vi "Add Header.vi"(8 "error in":errorcluster, 9 "value":string, 10 "header":string, 11 "http-client in":refnum<class "http-client.lvclass">) -> (0 "error out":errorcluster, 3 "http-client out":refnum<class "http-client.lvclass">)   [LabVIEW 2025, in "http-client.lvclass"]
uses:
  http-client.lvclass
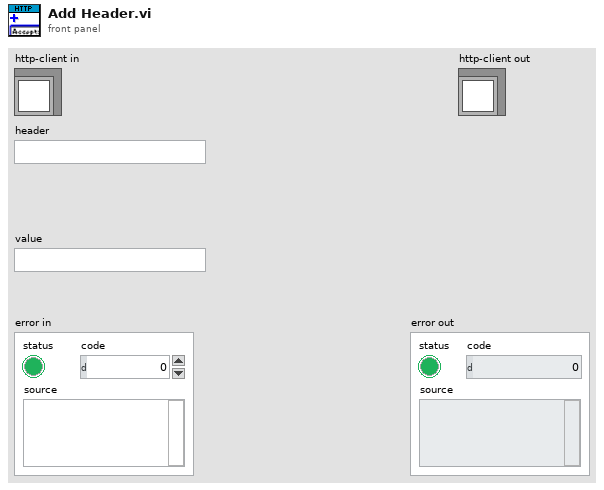
[diagram p1: front panel]
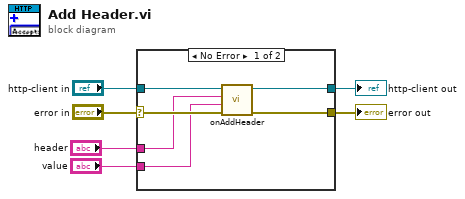
[diagram p0: block diagram]
diagram:
  n1 = case shown="No Error" "error in" {
    selector: "error in" -> [w9 w14]
    tunnel: [w10 w14] -> w5
    tunnel: [w11 w13] -> w3
    tunnel: "http-client in" -> [w12 w13]
    tunnel: "header" -> [w8 _]
    tunnel: "value" -> [w7 _]
    frame No Error {
      n2 = call-dynamic "onAddHeader.vi"("error in"=w9, "value"=w7, "header"=w8, "http-client in"=w12) -> ("error out"=w10:errorcluster, "http-client out"=w11:refnum<class "http-client.lvclass">)  [unwired: 6 in]
    }
    frame Error {
    }
  }
  "error out" <- w5
  "http-client out" <- w3
